vi "Calculate CoTan.vi"(10 "TimeConstant (sec)":dbl format="%13.5p", 11 "SamplePeriod (sec)":dbl format="%13.5p") -> (1 "In Range?":bool, 3 "C":dbl)   [LabVIEW 2023]
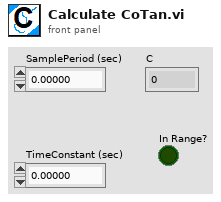
[diagram p1: front panel]
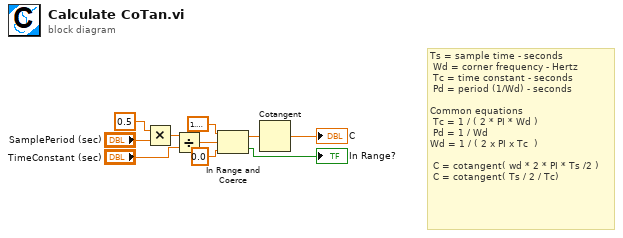
[diagram p0: block diagram]
diagram:
  # "Ts = sample time - seconds\n\tWd = corner frequency - Hertz\n\tTc = time constant - seconds\n\tPd = period (1/Wd) - seconds\n\nCommon equations\n\tTc = 1 / ( 2 * PI * Wd )\n\tPd = 1 / Wd\nWd = 1 / ( 2 x PI x Tc  )\n\t\n\tC = cotangent( wd * 2 * PI * Ts /2 )\n C = cotangent( Ts / 2 / Tc)"
  n1 = Multiply(x=0.5, y="SamplePeriod (sec)") -> (x*y=w4:dbl)
  n2 = Divide(x=w4, y="TimeConstant (sec)") -> (x/y=w7:dbl)
  n3 = In Range and Coerce(upper limit=1.5707963267948966, x=w7, lower limit=0.0) -> (coerced(x)=w10:dbl, In Range?=→"In Range?":bool)
  n4 = Cotangent(1:w10) -> (0:→"C":dbl)
